vi "ProcessRepository.vi"(0 "reference in":refnum<class "BKP-891 LCR Meter.lvclass">, 1 "Action(ReadRepository)":T1(ring), 5 "error in (no error)":errorcluster) -> (7 "QueueFromProcess":refnum<queue>, 9 "ProcessViRef":refnum<vi>, 11 "ProcessSyncQueue":refnum<queue>, 13 "EventFromProcess":refnum<user-event>, 14 "reference out":refnum<class "BKP-891 LCR Meter.lvclass">, 15 "EventsToProcess":refnum<user-event>, 17 "ProcessAlreadyStarted":bool, 19 "error out":errorcluster)   [LabVIEW 2020, in "BKP-891 LCR Meter.lvclass"]
uses:
  BKP-891 LCR Meter.lvclass
  Process.ctl
  BKP-891 LCR Meter.lvclass/BKP-891 LCR Meter.ctl
panel:
  # "Use this indicator for sending messages to the Process VI"
  # "These indicators are used by the process VIs"
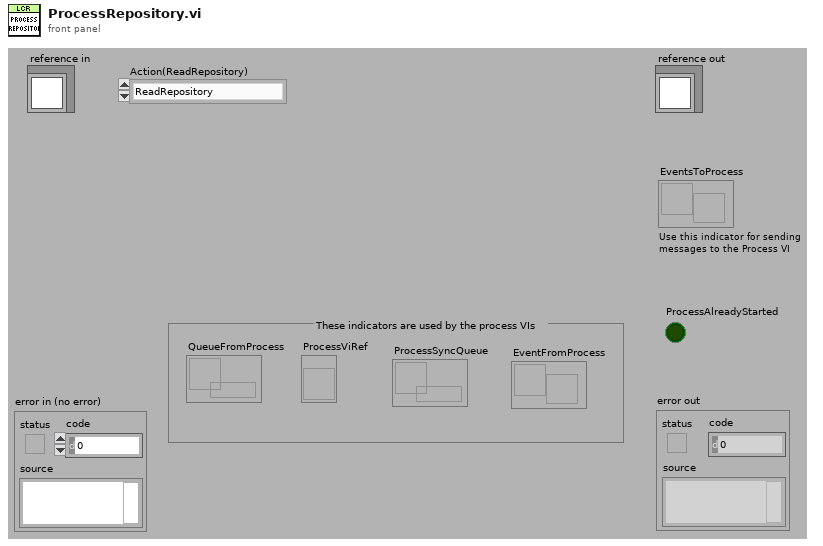
[diagram p1: front panel]
types:
  T1 = enum16{"ReadRepository", "CreateNew", "CreateOrLookUpExisting", "ReadRepositoryAndDestroy"}
  T2 = typedef "BKP-891 LCR Meter.lvclass/Process.ctl" = cluster{"EventsToProcess":refnum<user-event>, "EventFromProcess":refnum<user-event>, "ProcessSyncQueue":refnum<queue>, "ProcessViRef":refnum<vi>, "QueueFromProcess":refnum<queue>}
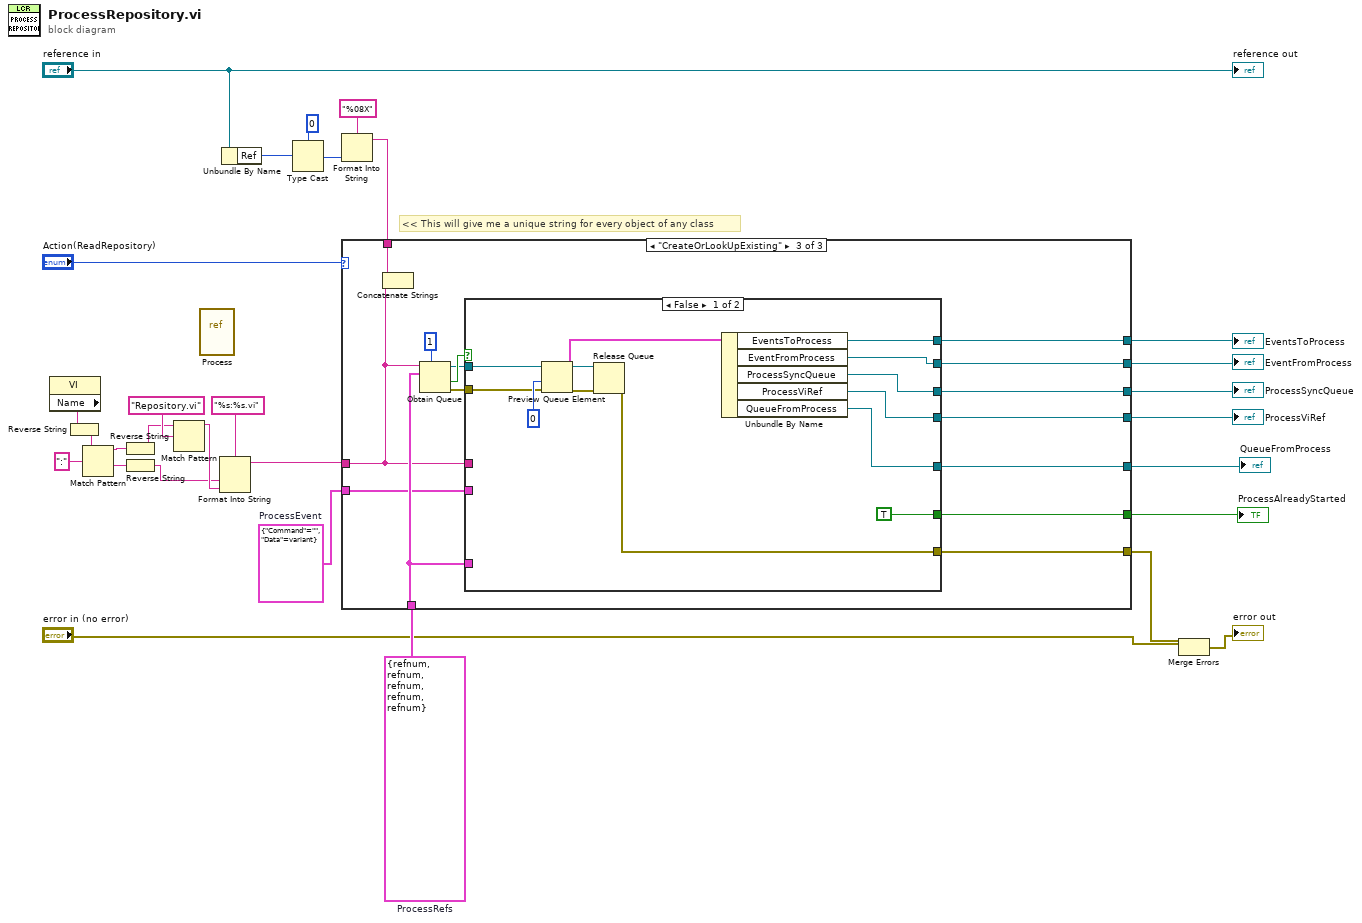
[diagram p0: block diagram]
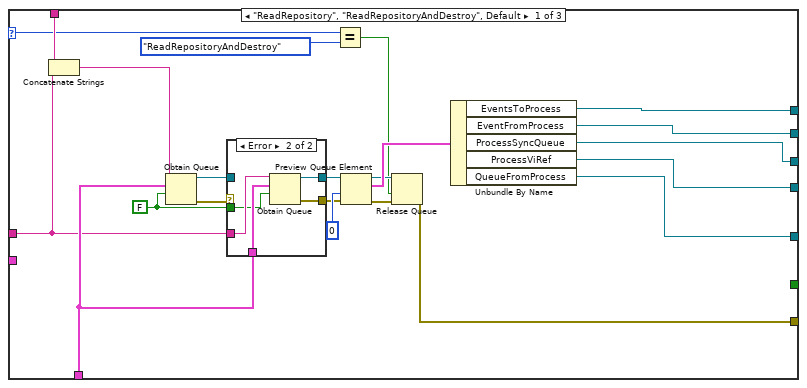
[diagram p2: hidden frame]
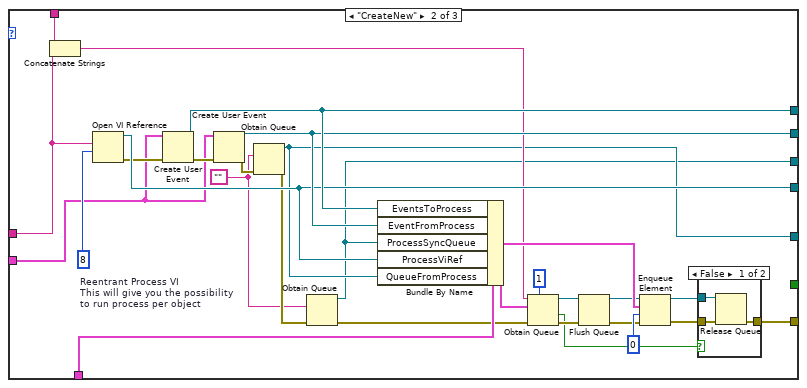
[diagram p4: hidden frame]
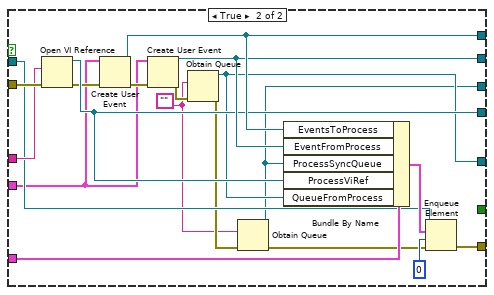
[diagram p6: hidden frame]
diagram:
  w13 = T2 {"EventsToProcess"=refnum, "EventFromProcess"=refnum, "ProcessSyncQueue"=refnum, "ProcessViRef"=refnum, "QueueFromProcess"=refnum}  # ProcessRefs
  w14 = cluster{"Command":string, "Data":variant} {"Command"="", "Data"=variant}  # ProcessEvent
  # "<< This will give me a unique string for every object of any class"
  n1 = property class="VI"() -> ("Name"=w20:string)  [unwired: 2 in, 2 out]
  n2 = Reverse String(1:w20) -> (0:w21:string)
  n3 = Match Pattern(string=w21, regular expression=":") -> (before substring=w25:string, after substring=w22:string)  [unwired: 1 in, 2 out]
  n4 = Reverse String(1:w25) -> (0:w26:string)
  n5 = Reverse String(1:w22) -> (0:w24:string)
  n6 = Match Pattern(string=w26, regular expression="Repository.vi") -> (before substring=w28:string)  [unwired: 1 in, 3 out]
  n7 = vi-ref "Process.vi"() -> ()  [unwired: 1 out]
  n8 = Format Into String(format string="%s:%s.vi", w24, w28) -> (resulting string=w3:string)  [unwired: 2 in, 1 out]
  n9 = Unbundle By Name("reference in") -> ("Ref"=w15:u32)
  n10 = Type Cast(type=u32 0, x=w15) -> (*(type *) &x=w18:u32)
  n11 = Format Into String(format string="%08X", w18) -> (resulting string=w5:string)  [unwired: 2 in, 1 out]
  n12 = case shown="\"CreateOrLookUpExisting\"" "Action(ReadRepository)" {
    selector: "Action(ReadRepository)" -> [w31 _ _]
    tunnel: [w47 w66 w103] -> w8
    tunnel: [w49 w86 w105] -> w6
    tunnel: [w48 w85 w104] -> w7
    tunnel: [w50 w84 w102] -> w9
    tunnel: w13 -> [w42 w76 w98]
    tunnel: w5 -> [w40 w75 w94]
    tunnel: [w33 w60 w101] -> w11
    tunnel: w3 -> [w39 w73 w91]
    tunnel: [_ _ w96] -> w10
    tunnel: w14 -> [_ w72 w93]
    tunnel: [w37 w70 w92] -> w1
    frame "ReadRepository", "ReadRepositoryAndDestroy", Default {
      w41 = FALSE ("create if not found? (T)")
      n13 = Concatenate Strings(w40, w39) -> (w38:string)
      n14 = Obtain Queue(name (unnamed)=w38, element data type=w42, create if not found? (T)=w41) -> (queue out=w44:refnum<queue>, error out=w46:errorcluster)  [unwired: 2 in, 1 out]
      n15 = case shown="Error" w46 {
        selector: w46 -> [w53 _]
        tunnel: [w53 w55] -> w45
        tunnel: w44 -> [w52 _]
        tunnel: [w52 w56] -> w43
        tunnel: w42 -> [_ w58]
        tunnel: w39 -> [_ w57]
        tunnel: w41 -> [_ w54]
        frame No Error {
        }
        frame Error {
          n16 = Obtain Queue(name (unnamed)=w57, element data type=w58, create if not found? (T)=w54) -> (queue out=w56:refnum<queue>, error out=w55:errorcluster)  [unwired: 2 in, 1 out]
        }
      }
      n17 = Equal?(x=w31, y=T1."ReadRepositoryAndDestroy") -> (x = y?=w30:bool)
      n18 = Preview Queue Element(queue=w43, timeout in ms (-1)=0, error in (no error)=w45) -> (queue out=w35:refnum<queue>, element=w36:T2, error out=w34:errorcluster)  [unwired: 1 out]
      n19 = Release Queue(queue=w35, force destroy? (F)=w30, error in (no error)=w34) -> (error out=w33:errorcluster)  [unwired: 2 out]
      n20 = Unbundle By Name(w36) -> ("EventsToProcess"=w49:refnum<user-event>, "EventFromProcess"=w48:refnum<user-event>, "ProcessSyncQueue"=w47:refnum<queue>, "ProcessViRef"=w50:refnum<vi>, "QueueFromProcess"=w37:refnum<queue>)
    }
    frame "CreateNew" {
      w67 = ""
      w81 = 8  # Reentrant Process VI This will give you the possibility to run process per object
      n21 = Concatenate Strings(w75, w73) -> (w74:string)
      n22 = Open VI Reference(vi path=w73, options=w81) -> (vi reference=w84:refnum<vi>, error out=w82:errorcluster)  [unwired: 4 in]
      n23 = Create User Event(user event datatype=w72, error in=w82) -> (user event=w86:refnum<user-event>, error out=w83:errorcluster)
      n24 = Create User Event(user event datatype=w72, error in=w83) -> (user event=w85:refnum<user-event>, error out=w71:errorcluster)
      n25 = Obtain Queue(element data type=w67, error in (no error)=w71) -> (queue out=w70:refnum<queue>, error out=w69:errorcluster)  [unwired: 3 in, 1 out]
      n26 = Obtain Queue(element data type=w67, error in (no error)=w69) -> (queue out=w66:refnum<queue>, error out=w68:errorcluster)  [unwired: 3 in, 1 out]
      n27 = Bundle By Name(cluster=w76, "EventsToProcess"=w86, "EventFromProcess"=w85, "ProcessSyncQueue"=w66, "ProcessViRef"=w84, "QueueFromProcess"=w70) -> (w79:T2)
      n28 = Obtain Queue(max queue size (-1, unlimited)=1, name (unnamed)=w74, element data type=w79, error in (no error)=w68) -> (queue out=w80:refnum<queue>, created new?=w59:bool, error out=w64:errorcluster)  [unwired: 1 in]
      n29 = Flush Queue(queue=w80, error in (no error)=w64) -> (queue out=w65:refnum<queue>, error out=w63:errorcluster)  [unwired: 1 out]
      n30 = Enqueue Element(queue=w65, element=w79, timeout in ms (-1)=0, error in (no error)=w63) -> (queue out=w61:refnum<queue>, error out=w62:errorcluster)  [unwired: 1 out]
      n31 = case shown="False" w59 {
        tunnel: w62 -> [w89 w90]
        tunnel: w61 -> [w88 _]
        tunnel: [w87 w90] -> w60
        frame False {
          n32 = Release Queue(queue=w88, error in (no error)=w89) -> (error out=w87:errorcluster)  [unwired: 1 in, 2 out]
        }
        frame True {
        }
      }
    }
    frame "CreateOrLookUpExisting" {
      n33 = Concatenate Strings(w94, w91) -> ()  [unwired: 1 out]
      n34 = Obtain Queue(max queue size (-1, unlimited)=1, name (unnamed)=w91, element data type=w98) -> (queue out=w99:refnum<queue>, created new?=w100:bool, error out=w97:errorcluster)  [unwired: 2 in]
      n35 = case shown="False" w100 {
        tunnel: [w118 w137] -> w105
        tunnel: [w117 w136] -> w104
        tunnel: [w116 w119] -> w103
        tunnel: [w115 w135] -> w102
        tunnel: [w106 w134] -> w101
        tunnel: w98 -> [_ w133]
        tunnel: w97 -> [w112 w128]
        tunnel: w91 -> [_ w127]
        tunnel: w99 -> [w113 w126]
        tunnel: [TRUE _] -> w96
        tunnel: w93 -> [_ w125]
        tunnel: [w109 w123] -> w92
        frame False {
          n36 = Preview Queue Element(queue=w113, timeout in ms (-1)=0, error in (no error)=w112) -> (queue out=w108:refnum<queue>, element=w111:T2, error out=w107:errorcluster)  [unwired: 1 out]
          n37 = Release Queue(queue=w108, error in (no error)=w107) -> (error out=w106:errorcluster)  [unwired: 1 in, 2 out]
          n38 = Unbundle By Name(w111) -> ("EventsToProcess"=w118:refnum<user-event>, "EventFromProcess"=w117:refnum<user-event>, "ProcessSyncQueue"=w116:refnum<queue>, "ProcessViRef"=w115:refnum<vi>, "QueueFromProcess"=w109:refnum<queue>)
        }
        frame True {
          w120 = ""
          n39 = Open VI Reference(vi path=w127, error in (no error)=w128) -> (vi reference=w135:refnum<vi>, error out=w131:errorcluster)  [unwired: 4 in]
          n40 = Create User Event(user event datatype=w125, error in=w131) -> (user event=w137:refnum<user-event>, error out=w132:errorcluster)
          n41 = Create User Event(user event datatype=w125, error in=w132) -> (user event=w136:refnum<user-event>, error out=w124:errorcluster)
          n42 = Obtain Queue(element data type=w120, error in (no error)=w124) -> (queue out=w123:refnum<queue>, error out=w122:errorcluster)  [unwired: 3 in, 1 out]
          n43 = Obtain Queue(element data type=w120, error in (no error)=w122) -> (queue out=w119:refnum<queue>, error out=w121:errorcluster)  [unwired: 3 in, 1 out]
          n44 = Bundle By Name(cluster=w133, "EventsToProcess"=w137, "EventFromProcess"=w136, "ProcessSyncQueue"=w119, "ProcessViRef"=w135, "QueueFromProcess"=w123) -> (w130:T2)
          n45 = Enqueue Element(queue=w126, element=w130, timeout in ms (-1)=0, error in (no error)=w121) -> (error out=w134:errorcluster)  [unwired: 2 out]
        }
      }
    }
  }
  "ProcessSyncQueue" <- w8
  "EventsToProcess" <- w6
  "EventFromProcess" <- w7
  "ProcessViRef" <- w9
  "ProcessAlreadyStarted" <- w10
  "QueueFromProcess" <- w1
  n46 = Merge Errors("error in (no error)", w11) -> (→"error out":errorcluster)
  "reference out" <- "reference in"
